vi "20.4 Compute Depth Image.vi"() -> ()   [LabVIEW 2017]
uses:
  <vilib>/vision/Image Controls.llb/IMAQ Image.ctl
  <vilib>/vision/NI_Vision_Development_Module.lvlib
panel:
  out "Depth(cm):":dbl format="%#_2g"
  out "DImg":sgl[][](graph)
  out "Tip:":string
  in  "RC":bool
  out "Right":T1(plugin-control)
  out "Left":T1(plugin-control)
  in  "Calibrate":bool
  in  "Exit":bool
  out "ErrOut":errorcluster
  in  "ErrIn":errorcluster
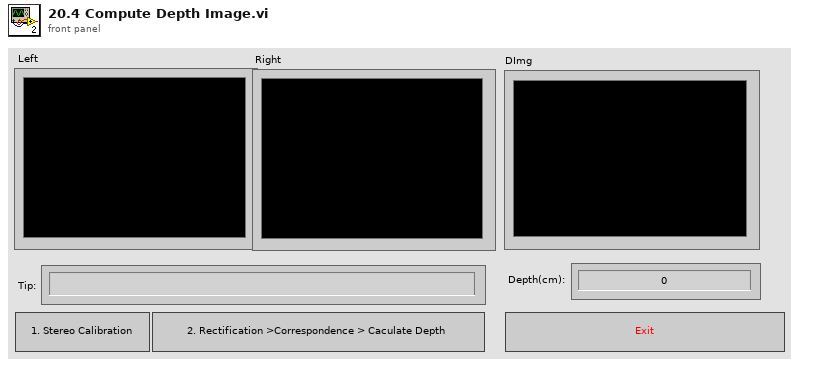
[diagram p1: front panel]
types:
  T1 = typedef "IMAQ Image.ctl" = refnum<image>
  T2 = cluster{"Number of Disparity":dbl, "Number of Disparity":dbl}
  T3 = enum8{"Enabled", "Disabled", "Disabled and Grayed Out"}
  T4 = typedef "LVPoint32TypeDef.ctl" = cluster{"Horizontal":i32, "Vertical":i32}
  T5 = typedef "IMAQ Binocular Stereo Session.ctl" = refnum<k1>
  T6 = cluster{"ImgR":T1, "ImgL":T1, "Path":path, "ImgD":T1, "Session":T5}
  T7 = typedef "Calibration Reference Points.ctl" = cluster{"Pixel Coordinates":cluster{"X":dbl, "Y":dbl}[], "Real World Coordinates":cluster{"X":dbl, "Y":dbl}[], "Unit":T8, "Image Size":cluster{"X":u32, "Y":u32}}
  T8 = typedef "Image Unit" = enum32{"Undefined", "Angström", "Micrometer", "Millimeter", "Centimeter", "Meter", "Kilometer", "Microinch", "Inch", "Feet", "Nautical miles", "Standard miles", "Steps"}
  T9 = typedef "Image Type" = u32
  T10 = cluster{"Method":u16, "Window Size":dbl, "Minimum Disparity":dbl, "Number of Disparity":dbl, "P1":dbl, "P2":dbl, "Full DP":bool, "Max Left Right Disparity":dbl, "Subpixel":bool, "Invalid Disparity Replace Value":dbl}
  T11 = cluster{"Texture Threshold":dbl, "Uniqueness Ratio":dbl, "Speckle Window Size":dbl, "Speckle Range":dbl}
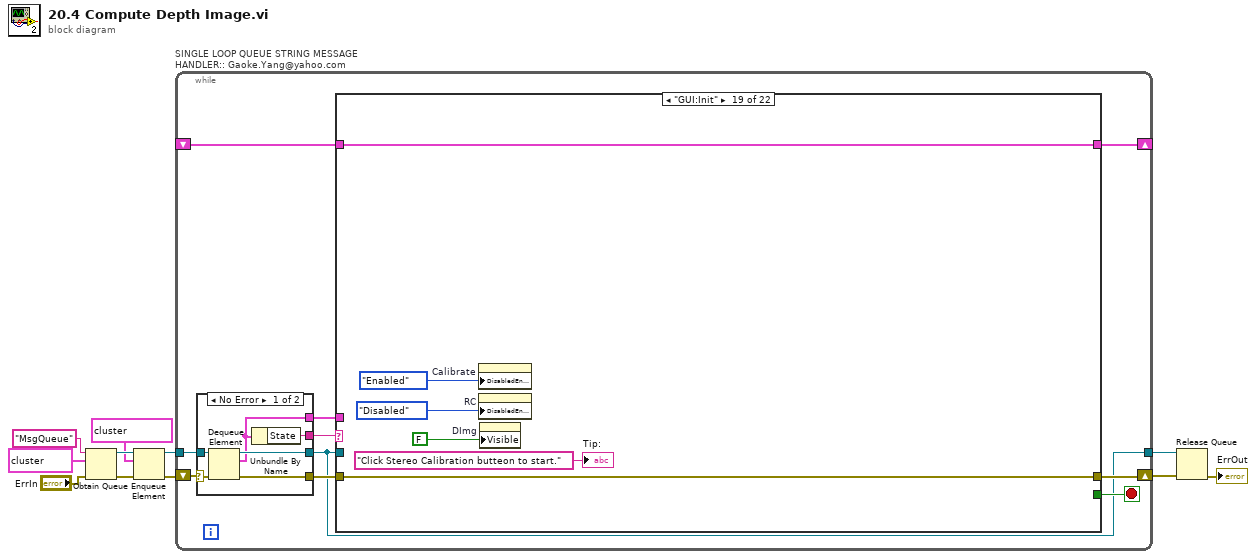
[diagram p0: block diagram]
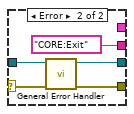
[diagram p2: hidden frame]
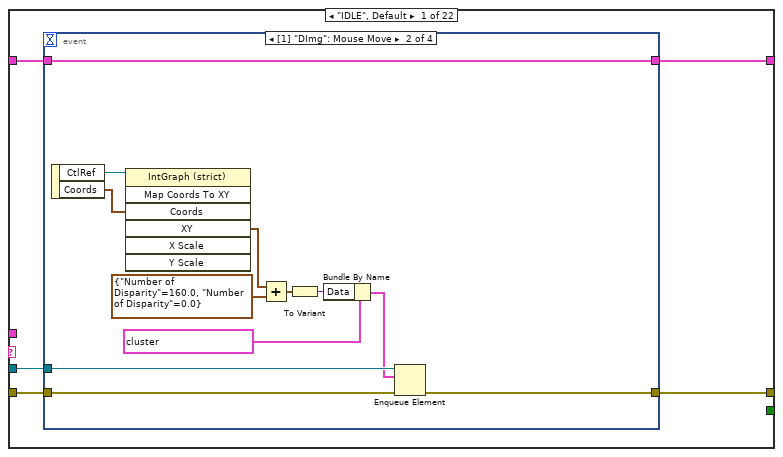
[diagram p3: hidden frame]
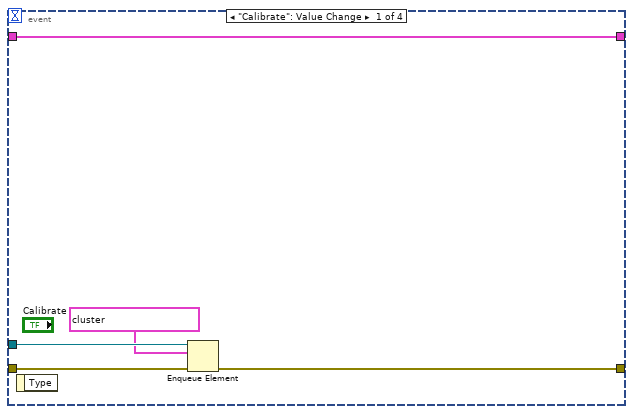
[diagram p4: hidden frame]
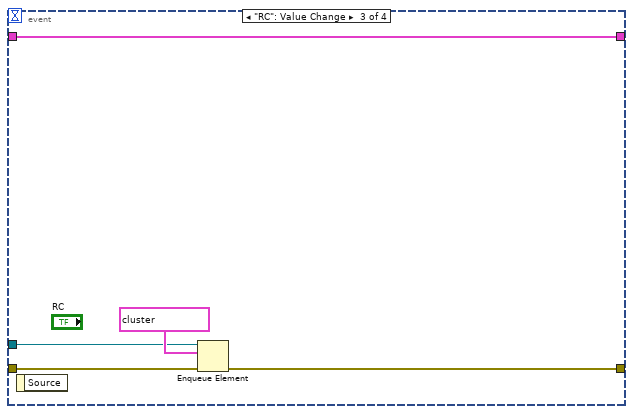
[diagram p5: hidden frame]
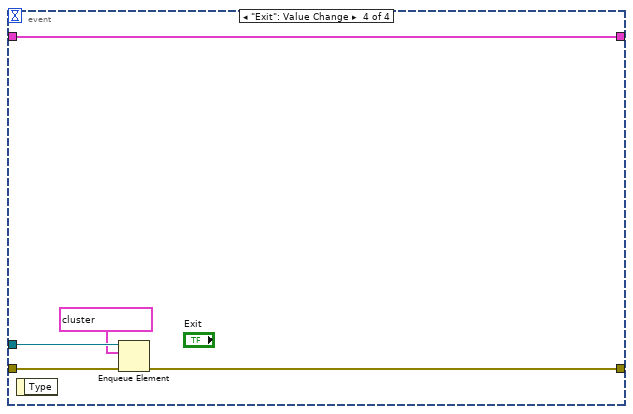
[diagram p6: hidden frame]
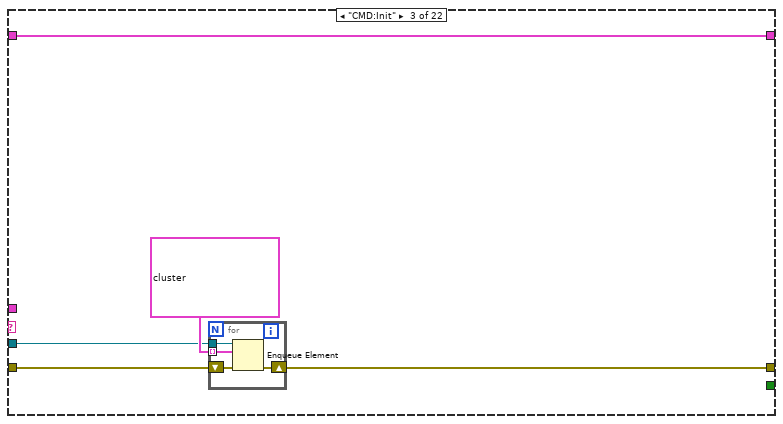
[diagram p8: hidden frame]
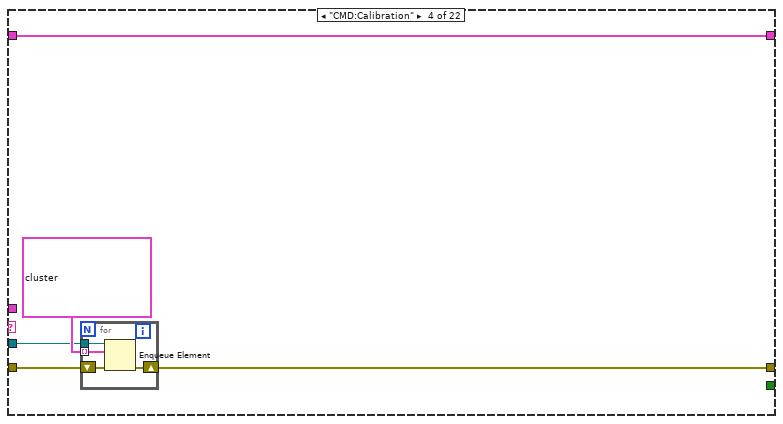
[diagram p9: hidden frame]
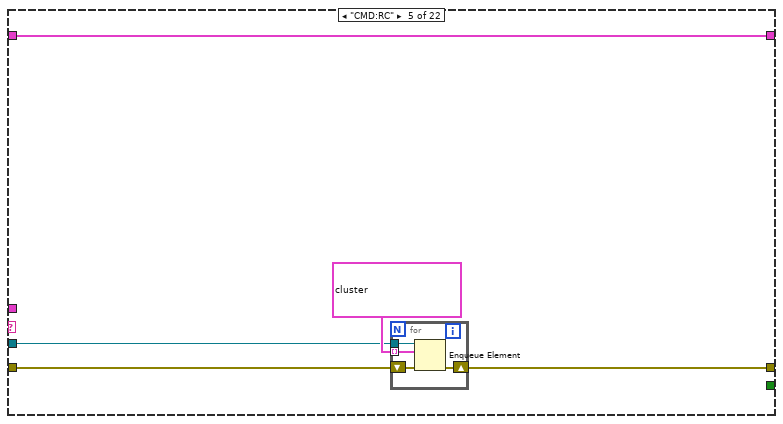
[diagram p10: hidden frame]
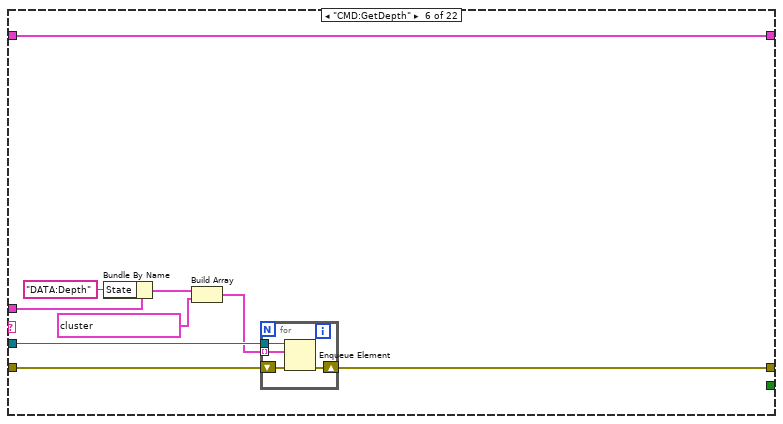
[diagram p11: hidden frame]
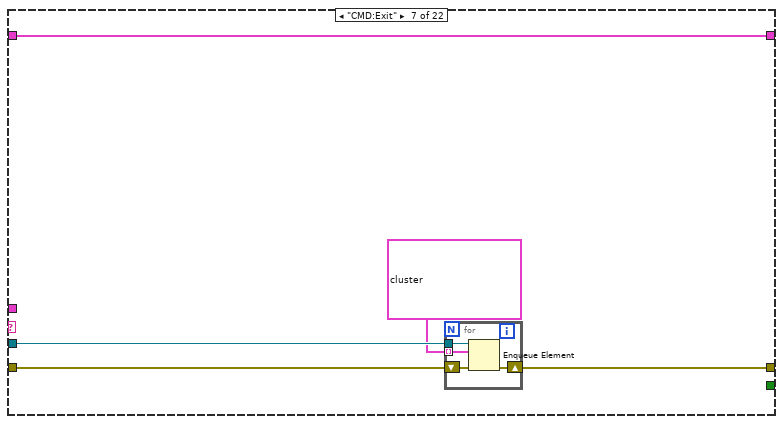
[diagram p12: hidden frame]
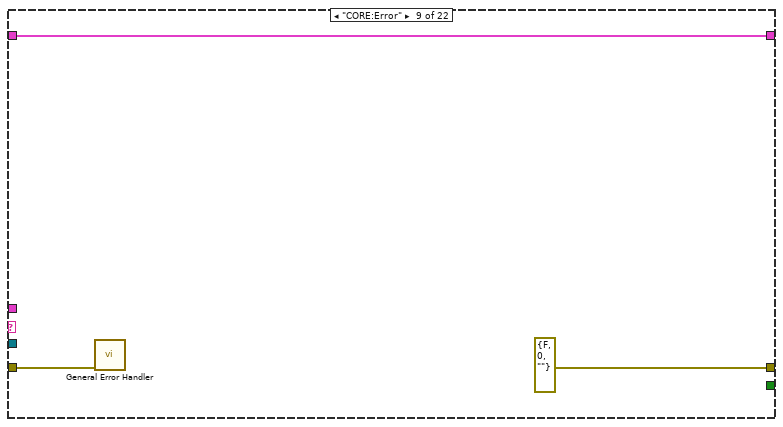
[diagram p14: hidden frame]
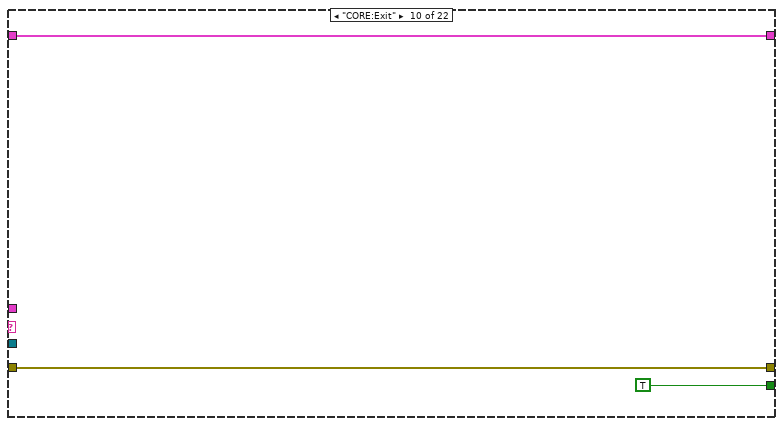
[diagram p15: hidden frame]
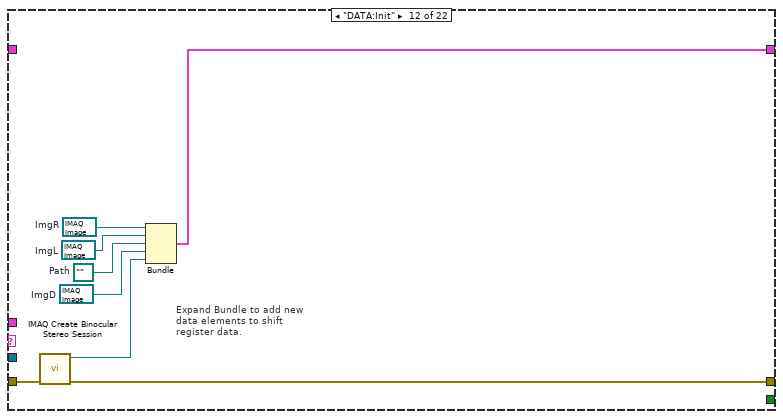
[diagram p17: hidden frame]
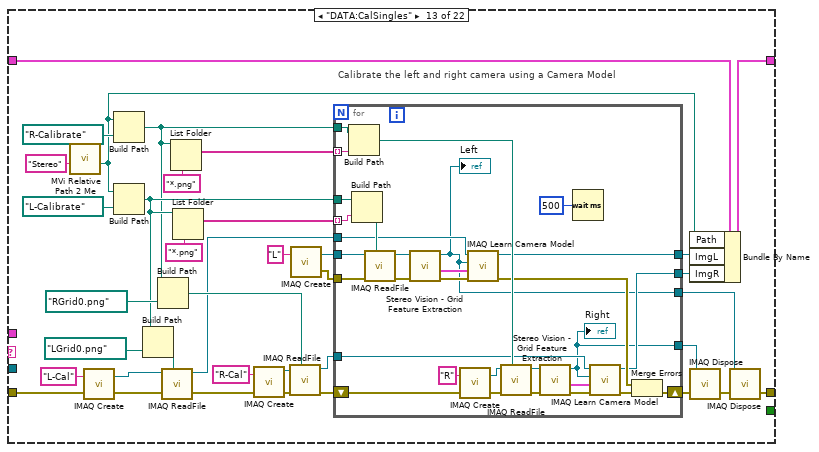
[diagram p18: hidden frame]
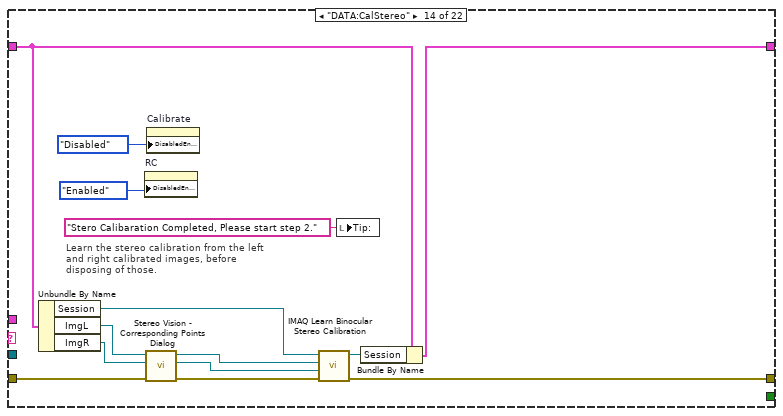
[diagram p19: hidden frame]
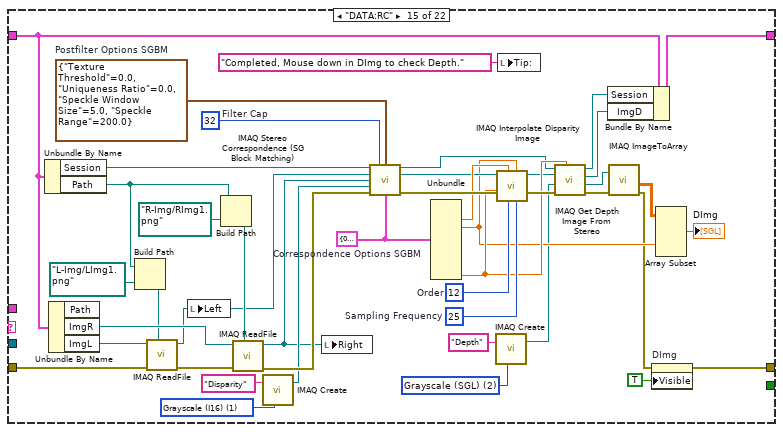
[diagram p20: hidden frame]
diagram:
  n1 = Obtain Queue(name (unnamed)="MsgQueue", element data type=cluster{"Data":variant, "State":string} {"Data"=variant, "State"="IDLE"} ("Queue Data"), error in (no error)="ErrIn") -> (queue out=w10:refnum<queue>, error out=w9:errorcluster)  [unwired: 2 in, 1 out]
  n2 = Enqueue Element(queue=w10, element=cluster{"Data":variant, "State":string} {"Data"=variant, "State"="CMD:Init"} ("Queue Data"), error in (no error)=w9) -> (queue out=w4:refnum<queue>, error out=w3:errorcluster)  [unwired: 1 in, 1 out]
  n3 = while "SINGLE LOOP QUEUE STRING MESSAGE HANDLER:: Gaoke.Yang@yahoo.com" {
    shift-right: [w20] -> w8
    shift-left: w3 -> [w18]
    tunnel: w4 -> [w19]
    tunnel: [w16] -> w7
    shift-right: [w15] -> _
    shift-left: _ -> [w13]
    stop <- w21 stop-if-true
    n4 = case shown="No Error" w18 {
      selector: w18 -> [w26 w31]
      tunnel: w19 -> [w27 w30]
      tunnel: [w25 w30] -> w16
      tunnel: [w24 w29] -> w17
      tunnel: [w23 "CORE:Exit" ("State")] -> w12
      tunnel: [w22 _] -> w14
      frame No Error {
        n5 = Dequeue Element(queue=w27, error in (no error)=w26) -> (queue out=w25:refnum<queue>, element=w22:cluster{"Data":variant, "State":string}, error out=w24:errorcluster)  [unwired: 1 in, 1 out]
        n6 = Unbundle By Name(w22) -> ("State"=w23:string)
      }
      frame Error {
        n7 = call <vilib>:"General Error Handler.vi"("error in (no error)"=w31) -> ("error out"=w29:errorcluster)  [unwired: 10 in, 4 out]
      }
    }
    n8 = case shown="\"GUI:Init\"" w12 {
      tunnel: [_ _ _ _ _ _ _ _ _ TRUE _ _ _ _ _ _ _ _ _ _ _ _] -> w21
      tunnel: w17 -> [w36 w65 w70 w79 w88 w101 w110 w116 w119 w121 w124 w127 w161 w213 w257 w267 w279 w283 w289 w291 w293 w295]
      tunnel: [w34 w65 w69 w78 w87 w100 w109 w116 errorcluster {"status"=FALSE, "code"=0, "source"=""} ("error out") w121 w124 w126 w141 w210 w214 w272 w274 w283 w289 w291 w293 w295] -> w20
      tunnel: w16 -> [w35 _ w67 w76 w85 w99 w108 _ _ _ _ _ _ _ _ _ _ _ _ _ _ _]
      tunnel: [w32 w64 w66 w75 w84 w98 w107 w115 w117 w120 w123 w132 w143 w201 w221 w259 w281 w282 w288 w290 w292 w294] -> w15
      tunnel: w14 -> [_ _ _ _ _ w97 _ _ _ _ _ _ _ _ _ w270 _ _ _ _ _ _]
      tunnel: w13 -> [w33 w64 w66 w75 w84 w98 w107 w115 w117 w120 w123 _ w169 w204 w222 w262 w281 w282 w288 w290 w292 w294]
      frame "IDLE", Default {
        n9 = event shown="[1] \"DImg\": Mouse Move" {
          selector: _ -> [_ _ _ _]
          dyn-events: _ -> [_ _ _ _]
          timeout: _ -> [_ _ _ _]
          tunnel: w36 -> [w41 w49 w56 w62]
          tunnel: w35 -> [w40 w48 w57 w63]
          tunnel: [w39 w47 w55 w61] -> w34
          tunnel: [w38 w42 w54 w59] -> w32
          tunnel: w33 -> [w38 w42 w54 w59]
          event "Calibrate": Value Change {
            n10 = event-data() -> ()  [unwired: 1 in, 1 out]
            n11 = Enqueue Element(queue=w40, element=cluster{"Data":variant, "name (unnamed)":string} {"Data"=variant, "name (unnamed)"="CMD:Calibration"} ("Queue Data"), error in (no error)=w41) -> (error out=w39:errorcluster)  [unwired: 1 in, 2 out]
          }
          event "DImg": Mouse Move {
            n12 = event-data() -> ("CtlRef"=w53:refnum<vi>, "Coords"=w52:T4)  [unwired: 1 in]
            n13 = invoke class="IntGraph (strict)" method="Map Coords To XY"(reference=w53, "Coords"=w52) -> ("XY"=w51:cluster{"X":dbl, "Y":dbl})  [unwired: 5 in, 6 out]
            n14 = Add(x=w51, y=T2 {"Number of Disparity"=160.0, "Number of Disparity"=0.0} ("output cluster")) -> (x+y=w44:cluster{dbl, dbl})
            n15 = To Variant(anything=w44) -> (Variant=w43:variant)
            n16 = Bundle By Name(cluster=cluster{"Data":variant, "name (unnamed)":string} {"Data"=variant, "name (unnamed)"="CMD:GetDepth"} ("Queue Data"), "Data"=w43) -> (w45:cluster{"Data":variant, "name (unnamed)":string})
            n17 = Enqueue Element(queue=w48, element=w45, error in (no error)=w49) -> (error out=w47:errorcluster)  [unwired: 1 in, 2 out]
          }
          event "RC": Value Change {
            n18 = event-data() -> ()  [unwired: 1 in, 1 out]
            n19 = Enqueue Element(queue=w57, element=cluster{"Data":variant, "name (unnamed)":string} {"Data"=variant, "name (unnamed)"="CMD:RC"} ("Queue Data"), error in (no error)=w56) -> (error out=w55:errorcluster)  [unwired: 1 in, 2 out]
          }
          event "Exit": Value Change {
            n20 = event-data() -> ()  [unwired: 1 in, 1 out]
            n21 = Enqueue Element(queue=w63, element=cluster{"Data":variant, "State":string} {"Data"=variant, "State"="CORE:Exit"} ("Queue Data"), error in (no error)=w62) -> (error out=w61:errorcluster)  [unwired: 1 in, 2 out]
          }
        }
      }
      frame "----------- CMD -----------" {
        # "Seperator Case"
      }
      frame "CMD:Init" {
        n22 = for {
          tunnel: w67 -> [w72]
          shift-right: [w73] -> w69
          shift-left: w70 -> [w74]
          tunnel: cluster{"Data":variant, "State":string}[] [{"Data"=variant, "State"="DATA:Init"}, {"Data"=variant, "State"="GUI:Init"}, {"Data"=variant, "State"="IDLE"}] -> [w71] mode=indexing
          n23 = Enqueue Element(queue=w72, element=w71, error in (no error)=w74) -> (error out=w73:errorcluster)  [unwired: 1 in, 2 out]
        }
      }
      frame "CMD:Calibration" {
        n24 = for {
          tunnel: w76 -> [w81]
          shift-right: [w82] -> w78
          shift-left: w79 -> [w83]
          tunnel: cluster{"Data":variant, "State":string}[] [{"Data"=variant, "State"="DATA:CalSingles"}, {"Data"=variant, "State"="DATA:CalStereo"}, {"Data"=variant, "State"="IDLE"}] -> [w80] mode=indexing
          n25 = Enqueue Element(queue=w81, element=w80, error in (no error)=w83) -> (error out=w82:errorcluster)  [unwired: 1 in, 2 out]
        }
      }
      frame "CMD:RC" {
        n26 = for {
          tunnel: w85 -> [w90]
          shift-right: [w91] -> w87
          shift-left: w88 -> [w92]
          tunnel: cluster{"Data":variant, "State":string}[] [{"Data"=variant, "State"="DATA:RC"}, {"Data"=variant, "State"="IDLE"}] -> [w89] mode=indexing
          n27 = Enqueue Element(queue=w90, element=w89, error in (no error)=w92) -> (error out=w91:errorcluster)  [unwired: 1 in, 2 out]
        }
      }
      frame "CMD:GetDepth" {
        n28 = Bundle By Name(cluster=w97, "State"="DATA:Depth") -> (w95:cluster{"Data":variant, "State":string})
        n29 = Build Array(w95, cluster{"Data":variant, "State":string} {"Data"=variant, "State"="IDLE"} ("Queue Data")) -> (w93:cluster{"Data":variant, "State":string}[])
        n30 = for {
          tunnel: w99 -> [w103]
          shift-right: [w104] -> w100
          shift-left: w101 -> [w105]
          tunnel: w93 -> [w102] mode=indexing
          n31 = Enqueue Element(queue=w103, element=w102, error in (no error)=w105) -> (error out=w104:errorcluster)  [unwired: 1 in, 2 out]
        }
      }
      frame "CMD:Exit" {
        n32 = for {
          tunnel: w108 -> [w112]
          shift-right: [w113] -> w109
          shift-left: w110 -> [w114]
          tunnel: cluster{"Data":variant, "State":string}[] [{"Data"=variant, "State"="GUI:FP"}, {"Data"=variant, "State"="DATA:CleanUp"}, {"Data"=variant, "State"="CORE:Exit"}, {"Data"=variant, "State"="GUI:FP"}] -> [w111] mode=indexing
          n33 = Enqueue Element(queue=w112, element=w111, error in (no error)=w114) -> (error out=w113:errorcluster)  [unwired: 1 in, 2 out]
        }
      }
      frame "----------- CORE -----------" {
        # "Seperator Case"
      }
      frame "CORE:Error" {
        n34 = call <vilib>:"General Error Handler.vi"("error in (no error)"=w119) -> ()  [unwired: 10 in, 5 out]
      }
      frame "CORE:Exit" {
      }
      frame "----------- DATA -----------" {
        # "Seperator Case"
      }
      frame "DATA:Init" {
        w128 = T1 refnum  # ImgD
        w129 = path ""  # Path
        w131 = T1 refnum  # ImgR
        w130 = T1 refnum  # ImgL
        # "Expand Bundle to add new data elements to shift register data."
        n35 = call "IMAQ Create Binocular Stereo Session"("error in (no error)"=w127) -> ("error out"=w126:errorcluster, "Session"=w125:T5)  [unwired: 9 out]
        n36 = Bundle("ImgR"=w131, "ImgL"=w130, "Path"=w129, "ImgD"=w128, "Session"=w125) -> (w132:T6)  [unwired: 1 in]
      }
      frame "DATA:CalSingles" {
        # "Calibrate the left and right camera using a Camera Model"
        n37 = call "MVi Relative Path 2 Me.vi"("Relative Path"="Stereo") -> ("Appended Dir"=w133:path)  [unwired: 5 in, 1 out]
        n38 = call "IMAQ Create"("Image Name"="L-Cal", "error in (no error)"=w161) -> ("New Image"=w158:T1, "error out"=w160:errorcluster)  [unwired: 3 in]
        n39 = Build Path(base path=w133, name or relative path=path "R-Calibrate" ("appended path")) -> (appended path=w134:path)
        n40 = Build Path(base path=w133, name or relative path=path "L-Calibrate" ("appended path")) -> (appended path=w135:path)
        n41 = Build Path(base path=w135, name or relative path=path "LGrid0.png" ("appended path")) -> (appended path=w155:path)
        n42 = Build Path(base path=w134, name or relative path=path "RGrid0.png" ("appended path")) -> (appended path=w153:path)
        n43 = call "IMAQ ReadFile"("File Path"=w155, "error in (no error)"=w160, "Image"=w158) -> ("error out"=w159:errorcluster, "Image Out"=w150:T1)  [unwired: 4 in, 3 out]
        n44 = List Folder(path=w134, pattern="*.png") -> (filenames=w148:string[])  [unwired: 2 in, 3 out]
        n45 = List Folder(path=w135, pattern="*.png") -> (filenames=w147:string[])  [unwired: 2 in, 3 out]
        n46 = call "IMAQ Create"("Image Name"="R-Cal", "error in (no error)"=w159) -> ("New Image"=w151:T1, "error out"=w154:errorcluster)  [unwired: 3 in]
        n47 = call "IMAQ ReadFile"("File Path"=w153, "error in (no error)"=w154, "Image"=w151) -> ("error out"=w149:errorcluster, "Image Out"=w152:T1)  [unwired: 4 in, 3 out]
        n48 = call "IMAQ Create"("Image Name"="L") -> ("New Image"=w145:T1, "error out"=w144:errorcluster)  [unwired: 4 in]
        n49 = for {
          tunnel: w152 -> [w177]
          tunnel: w150 -> [w178]
          shift-right: [w183] -> w142
          shift-left: w149 -> [w181]
          tunnel: w148 -> [w196] mode=indexing
          tunnel: w147 -> [w198] mode=indexing
          tunnel: w135 -> [w199]
          tunnel: w134 -> [w195]
          tunnel: w145 -> [w180]
          tunnel: w144 -> [w179]
          tunnel: [w172] -> w139
          tunnel: [w174] -> w138
          tunnel: [w171] -> w137
          tunnel: [w170] -> w136
          n50 = Build Path(base path=w195, name or relative path=w196) -> (appended path=w194:path)
          n51 = Build Path(base path=w199, name or relative path=w198) -> (appended path=w197:path)
          n52 = call "IMAQ ReadFile"("File Path"=w197, "error in (no error)"=w179, "Image"=w180) -> ("error out"=w190:errorcluster, "Image Out"=w189:T1)  [unwired: 4 in, 3 out]
          n53 = call "Stereo Vision - Grid Feature Extraction.vi"("error in (no error)"=w190, "Image in"=w189) -> ("error out"=w188:errorcluster, "Reference Points"=w176:T7, "Image (dup)"=w171:T1)  [unwired: 7 in]
          "Left" <- w171
          n54 = call "IMAQ Create"("Image Name"="R", "error in (no error)"=w181) -> ("New Image"=w191:T1, "error out"=w192:errorcluster)  [unwired: 3 in]
          n55 = call "IMAQ Learn Camera Model"("error in (no error)"=w188, "Reference Points"=w176, "Image"=w171, "Calibration Template Image"=w178) -> ("error out"=w182:errorcluster, "Calibration Template Image Out"=w172:T1)  [unwired: 2 in, 4 out]
          n56 = call "IMAQ ReadFile"("File Path"=w194, "error in (no error)"=w192, "Image"=w191) -> ("error out"=w187:errorcluster, "Image Out"=w186:T1)  [unwired: 4 in, 3 out]
          n57 = call "Stereo Vision - Grid Feature Extraction.vi"("error in (no error)"=w187, "Image in"=w186) -> ("error out"=w185:errorcluster, "Reference Points"=w175:T7, "Image (dup)"=w170:T1)  [unwired: 7 in]
          "Right" <- w170
          n58 = Wait (ms)(milliseconds to wait=u32 500) -> ()  [unwired: 1 out]
          n59 = call "IMAQ Learn Camera Model"("error in (no error)"=w185, "Reference Points"=w175, "Image"=w170, "Calibration Template Image"=w177) -> ("error out"=w184:errorcluster, "Calibration Template Image Out"=w174:T1)  [unwired: 2 in, 4 out]
          n60 = Merge Errors(w182, w184) -> (w183:errorcluster)
        }
        n61 = Bundle By Name(cluster=w169, "Path"=w133, "ImgL"=w139, "ImgR"=w138) -> (w143:T6)
        n62 = call "IMAQ Dispose"("Image"=w136, "error in (no error)"=w142) -> ("error out"=w140:errorcluster)  [unwired: 4 in]
        n63 = call "IMAQ Dispose"("Image"=w137, "error in (no error)"=w140) -> ("error out"=w141:errorcluster)  [unwired: 4 in]
      }
      frame "DATA:CalStereo" {
        # "Learn the stereo calibration from the left and right calibrated images, before disposing of those."
        n64 = Unbundle By Name(w204) -> ("Session"=w202:T5, "ImgL"=w212:T1, "ImgR"=w211:T1)
        n65 = property on="RC" class="Bool"("DisabledEnum"=T3."Enabled" ("Disabled")) -> ()  [unwired: 2 in, 2 out]
        n66 = call "Stereo Vision - Corresponding Points Dialog.vi"("error in (no error)"=w213, "Right Image in"=w211, "Left Image in"=w212) -> ("error out"=w203:errorcluster, "Right Image out"=w208:T1, "Left Image out"=w209:T1)  [unwired: 6 in]
        n67 = property on="Calibrate" class="Bool"("DisabledEnum"=T3."Disabled" ("Disabled")) -> ()  [unwired: 2 in, 2 out]
        n68 = call "IMAQ Learn Binocular Stereo Calibration"("error in (no error)"=w203, "Right Calibration Template"=w208, "Left Calibration Template"=w209, "Binocular Stereo Session"=w202) -> ("error out"=w210:errorcluster, "Binocular Stereo Session (dup)"=w200:T5)  [unwired: 1 in, 5 out]
        n69 = local write "Tip:"("Stero Calibaration Completed, Please start step 2." ("Tip:")) -> ()
        n70 = Bundle By Name(cluster=w204, "Session"=w200) -> (w201:T6)
      }
      frame "DATA:RC" {
        w223 = T9 2 items=["Grayscale (U8)", "Grayscale (I16)", "Grayscale (SGL)", "Complex (CSG)", "RGB (U32)", "HSL (U32)", "RGB (U64)", "Grayscale (U16)"] ("Image Type")
        w224 = T9 1 items=["Grayscale (U8)", "Grayscale (I16)", "Grayscale (SGL)", "Complex (CSG)", "RGB (U32)", "HSL (U32)", "RGB (U64)", "Grayscale (U16)"] ("Image Type")
        w242 = 25  # Sampling Frequency
        w243 = 12  # Order
        w240 = T10 {"Method"=0, "Window Size"=25.0, "Minimum Disparity"=0.0, "Number of Disparity"=160.0, "P1"=100.0, "P2"=500.0, "Full DP"=FALSE, "Max Left Right Disparity"=5.0, "Subpixel"=TRUE, "Invalid Disparity Replace Value"=-16.0}  # Correspondence Options SGBM
        w245 = u32 32  # Filter Cap
        w244 = T11 {"Texture Threshold"=0.0, "Uniqueness Ratio"=0.0, "Speckle Window Size"=5.0, "Speckle Range"=200.0}  # Postfilter Options SGBM
        n71 = Unbundle By Name(w222) -> ("Session"=w219:T5, "Path"=w251:path)
        n72 = Unbundle By Name(w222) -> ("ImgR"=w254:T1, "ImgL"=w255:T1)  [unwired: 1 out]
        n73 = Build Path(base path=w251, name or relative path=path "L-Img/LImg1.png" ("appended path")) -> (appended path=w252:path)
        n74 = call "IMAQ ReadFile"("File Path"=w252, "error in (no error)"=w257, "Image"=w255) -> ("error out"=w256:errorcluster, "Image Out"=w227:T1)  [unwired: 2 in, 5 out]
        n75 = local write "Left"(w227) -> ()
        n76 = Build Path(base path=w251, name or relative path=path "R-Img/RImg1.png" ("appended path")) -> (appended path=w249:path)
        n77 = call "IMAQ ReadFile"("File Path"=w249, "error in (no error)"=w256, "Image"=w254) -> ("error out"=w248:errorcluster, "Image Out"=w226:T1)  [unwired: 2 in, 5 out]
        n78 = call "IMAQ Create"("Image Name"="Disparity", "Image Type"=w224) -> ("New Image"=w246:T1)  [unwired: 3 in, 1 out]
        n79 = local write "Right"(w226) -> ()
        n80 = call "IMAQ Stereo Correspondence (SG Block Matching)"("Binocular Stereo Session"=w219, "Filter Cap"=w245, "Postfilter Options"=w244, "Left Image In"=w227, "Right Image In"=w226, "Disparity Image In"=w246, "error in (no error)"=w248, "Correspondence Options"=w240) -> ("Binocular Stereo Session (dup)"=w218:T5, "Disparity Image Out"=w237:T1, "error out"=w241:errorcluster)  [unwired: 2 in, 3 out]
        n81 = Unbundle(w240) -> ("Minimum Disparity"=w239:dbl, "Number of Disparity"=w232:dbl, "Invalid Disparity Replace Value"=w236:dbl)  [unwired: 7 out]
        n82 = call "IMAQ Create"("Image Name"="Depth", "Image Type"=w223) -> ("New Image"=w228:T1)  [unwired: 3 in, 1 out]
        n83 = call "IMAQ Interpolate Disparity Image"("Sampling Frequency"=w242, "Number of Disparities"=w232, "Order"=w243, "Minimum Disparity"=w239, "error in (no error)"=w241, "Invalid Disparity Value"=w236, "Image Src"=w237) -> ("error out"=w238:errorcluster, "Image Dst Out"=w230:T1)  [unwired: 1 in, 2 out]
        n84 = local write "Tip:"("Completed, Mouse down in DImg to check Depth." ("Tip:")) -> ()
        n85 = call "IMAQ Get Depth Image From Stereo"("Invalid Disparity Value"=w236, "error in (no error)"=w238, "Depth Image In"=w228, "Disparity Image"=w230, "Binocular Stereo Session"=w218) -> ("error out"=w235:errorcluster, "Depth Image Out"=w234:T1, "Disparity Image (duplicate)"=w220:T1, "Binocular Stereo Session (dup)"=w217:T5)  [unwired: 2 in, 1 out]
        n86 = Bundle By Name(cluster=w222, "Session"=w217, "ImgD"=w220) -> (w221:T6)
        n87 = call "IMAQ ImageToArray"("error in (no error)"=w235, "Image"=w234) -> ("Image Pixels (Float)"=w233:sgl[][], "error out"=w215:errorcluster)  [unwired: 1 in, 4 out]
        n88 = property on="DImg" class="IntGraph (strict)"(error in=w215, "Visible"=TRUE) -> (error out=w214:errorcluster)  [unwired: 1 in, 1 out]
        n89 = Array Subset(array=w233, index (col)=w232) -> (→"DImg":sgl[][])  [unwired: 3 in]
      }
      frame "DATA:Depth" {
        n90 = Unbundle By Name(w270) -> ("Data"=w269:variant)
        n91 = Unbundle By Name(w262) -> ("Session"=w261:T5, "ImgD"=w260:T1)
        n92 = Variant To Data(error in=w267, type=cluster{dbl, dbl} {0.0, 0.0} ("x+y"), Variant=w269) -> (data=w265:cluster{dbl, dbl}, error out=w266:errorcluster)
        n93 = call "IMAQ Convert Pixel To 3D Coordinates"("Binocular Stereo Session"=w261, "Disparity Image"=w260, "Pixel Coordinates"=w265, "error in (no error)"=w266, "Depth Control"=cluster{"Min Depth":dbl, "Max Depth":dbl} {"Min Depth"=25.0, "Max Depth"=40.0}) -> ("Binocular Stereo Session (dup)"=w258:T5, "Real World 3D Coordinates"=w264:cluster{"X":dbl, "Y":dbl, "Z":dbl}, "error out"=w272:errorcluster)  [unwired: 3 in, 5 out]
        n94 = Unbundle By Name(w264) -> ("Z"=→"Depth(cm):":dbl)
        n95 = Bundle By Name(cluster=w262, "Session"=w258) -> (w259:T6)
      }
      frame "DATA:CleanUp" {
        n96 = Unbundle By Name(w281) -> ("Session"=w273:T5, "ImgR"=w280:T1, "ImgL"=w277:T1)
        n97 = call "IMAQ Dispose"("Image"=w277, "error in (no error)"=w279) -> ("error out"=w278:errorcluster)  [unwired: 4 in]
        n98 = call "IMAQ Dispose"("All Images? (No)"=TRUE, "Image"=w280, "error in (no error)"=w278) -> ("error out"=w275:errorcluster)  [unwired: 3 in]
        n99 = call "IMAQ Dispose Binocular Stereo Session"("error in (no error)"=w275, "Binocular Stereo Session"=w273) -> ("error out"=w274:errorcluster)  [unwired: 9 in]
      }
      frame "----------- GUI -----------" {
        # "Seperator Case"
      }
      frame "GUI:Init" {
        n100 = property on="Calibrate" class="Bool"("DisabledEnum"=T3."Enabled" ("Disabled")) -> ()  [unwired: 2 in, 2 out]
        n101 = property on="RC" class="Bool"("DisabledEnum"=T3."Disabled" ("Disabled")) -> ()  [unwired: 2 in, 2 out]
        n102 = property on="DImg" class="IntGraph (strict)"("Visible"=FALSE) -> ()  [unwired: 2 in, 2 out]
        "Tip:" <- "Click Stereo Calibration butteon to start." ("Tip:")
      }
      frame "GUI:SetCusor" {
      }
      frame "GUI:FP" {
      }
      frame "----------- RESERVED -----------" {
        # "Seperator Case"
      }
    }
  }
  n103 = Release Queue(queue=w7, error in (no error)=w8) -> (error out=→"ErrOut":errorcluster)  [unwired: 1 in, 2 out]
